vi "Load TCS mode.vi"(8 "error in (no error)":errorcluster, 10 "tcs mode":string, 11 "Acquisition in":refnum<class "Acquisition.lvclass">) -> (0 "error out":errorcluster, 3 "Acquisition out":refnum<class "Acquisition.lvclass">)   [LabVIEW 2018, in "Acquisition.lvclass"]
uses:
  Acquisition.lvclass
  Acquisition.lvclass/Acquisition.ctl
  Channel/Channel.lvclass
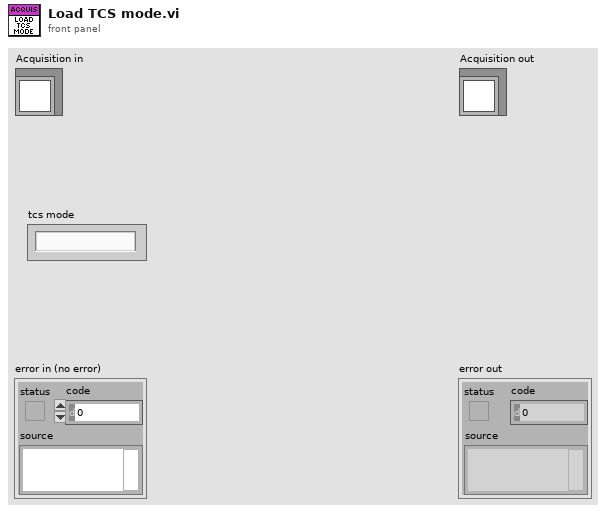
[diagram p1: front panel]
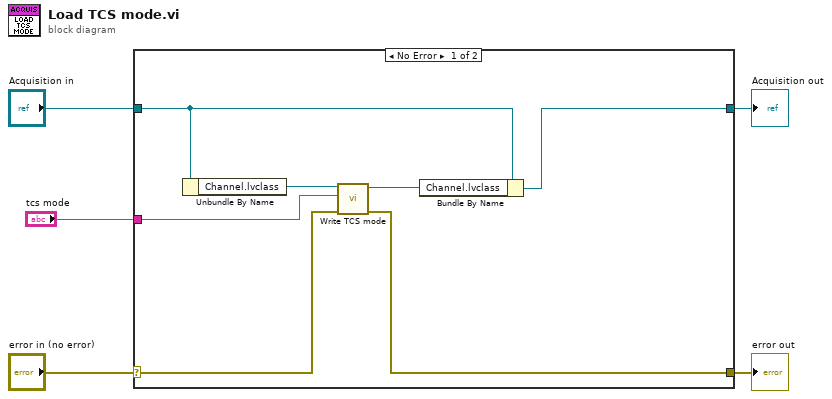
[diagram p0: block diagram]
diagram:
  n1 = case shown="No Error" "error in (no error)" {
    selector: "error in (no error)" -> [w7 w14]
    tunnel: [w6 w14] -> w4
    tunnel: [w9 w13] -> w2
    tunnel: "Acquisition in" -> [w10 w13]
    tunnel: "tcs mode" -> [w12 _]
    frame No Error {
      n2 = Unbundle By Name(w10) -> ("Channel.lvclass"=w11:refnum<class "Channel.lvclass">)
      n3 = call-dynamic "Write TCS mode.vi"("error in (no error)"=w7, "TCS mode"=w12, "Channel in"=w11) -> ("error out"=w6:errorcluster, "Channel out"=w8:refnum<class "Channel.lvclass">)  [unwired: 7 in]
      n4 = Bundle By Name(cluster=w10, "Channel.lvclass"=w8) -> (w9:refnum<class "Acquisition.lvclass">)
    }
    frame Error {
    }
  }
  "error out" <- w4
  "Acquisition out" <- w2
